vi "Triangular Egde Generator.vi"(7 "fattore":dbl=0.5, 8 "Sample values":dbl[](graph), 11 "Triangular edge":enum16{"Rising", "Falling"}(ring)=enum."Falling") -> (2 "Skew Triangular":dbl[](array[numeric]))   [LabVIEW 2014]
uses:
  <vilib>/imath/engines/lvmath2/RunTimeEngine/BuiltInFunctions/linramp/NIMS_linramp.vi
  <vilib>/imath/engines/lvmath2/RunTimeEngine/NodeEndStatement/NIMS_NodeEndStatement_Output.vi
  <instcachedir>/0/NIMS_NodeEndStatement_Output_53EC0D466D134D7ABD903AC30B43404B.lvgen/NIMS_NodeEndStatement_Output_53EC0D466D134D7ABD903AC30B43404B_005.vi
  <vilib>/imath/engines/lvmath2/RunTimeEngine/ErrorHandling/NIMS_Finalize Error.vi
  <vilib>/imath/engines/lvmath2/RunTimeEngine/BuiltInFunctions/max/1 input/NIMS_max(RV).vi
  <instcachedir>/0/NIMS_max(RV)_237633DB1D604D5BA7001287DF3C7957.lvgen/NIMS_max(RV)_237633DB1D604D5BA7001287DF3C7957_000.vi
  <vilib>/imath/engines/lvmath2/RunTimeEngine/ArithmeticOperatorToken/NIMS_ArithmeticOperator_times.vi
  <instcachedir>/0/NIMS_ArithmeticOperator_times_2EFF5B13FCA4492A81D59089AD809F54.lvgen/NIMS_ArithmeticOperator_times_2EFF5B13FCA4492A81D59089AD809F54_000.vi
  <vilib>/imathl/engines/lvmath/Functions/Error Handling/Create Error.vi
  <vilib>/imath/engines/lvmath2/RunTimeEngine/BuiltInFunctions/round/NIMS_round(DBL-V).vi
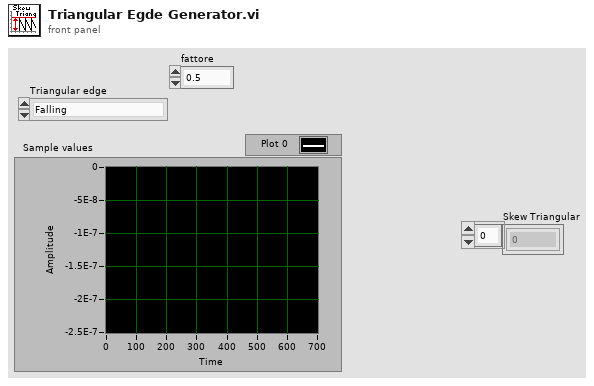
[diagram p1: front panel]
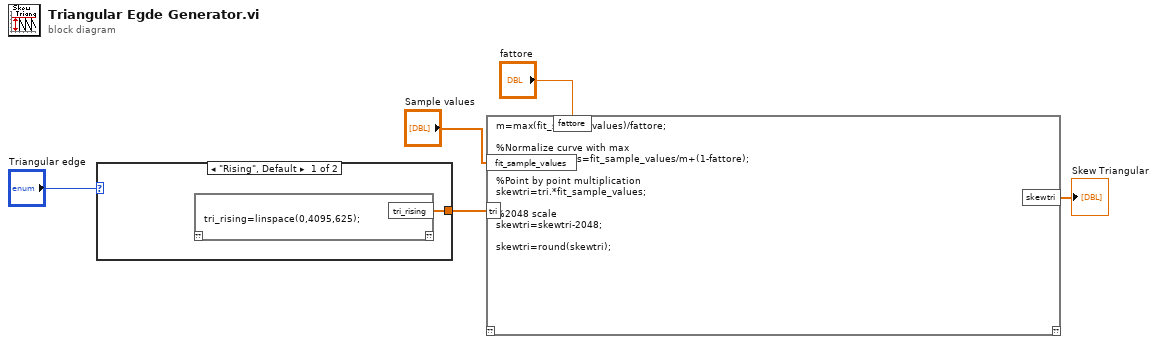
[diagram p0: block diagram]
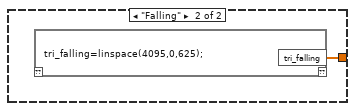
[diagram p2: hidden frame]
diagram:
  n1 = case shown="\"Rising\", Default" "Triangular edge" {
    tunnel: [w6 w26] -> w4
    frame "Rising", Default {
      n2 = mathscript code="tri_rising=linspace(0,4095,625);"() -> ("tri_rising"=w6:dbl[])  [unwired: 1 in, 1 out]
    }
    frame "Falling" {
      n3 = mathscript code="tri_falling=linspace(4095,0,625);"() -> ("tri_falling"=w26:dbl[])  [unwired: 1 in, 1 out]
    }
  }
  n4 = mathscript code="m=max(fit_sample_values)/fattore;\n\n%Normalize curve with max\nfit_sample_values=fit_sample_values/m+(1-fattore);\n\n%Point by point multiplication\nskewtri=tri.*fit_sample_values;\n\n%2048 scale\nskewtri=skewtri-2048;\n\nskewtri=round(skewtri);"("fit_sample_values"="Sample values", "tri"=w4, "fattore"="fattore") -> ("skewtri"=→"Skew Triangular":dbl[])  [unwired: 1 in, 1 out]
